vi "XNET Example IP Stack Config - Add Proxy Server Extended.vi"(0 "config in":string, 1 "forwarding destination address":string, 2 "forwarding destination port":u16, 5 "protocol":string(combo)="tcp", 7 "direction":string(combo)="outbound", 9 "listen port":u16, 11 "error in (no error)":errorcluster, 12 "listen address":string, 13 "forwarding source address":string, 14 "forwarding source port":u16) -> (4 "config out":string, 15 "error out":errorcluster)   [LabVIEW 2026]
doc: "This example subVI adds configuration for a single proxy server instance to an existing JSON configuration string for use with XNET IP Stack Create.vi. Configuration parameter definitions:\n\nprotocol: Protocol to use for the proxy server, which can be one of 1) tcp, 2) udp.\n\ndirection: Direction to use for the proxy server, which can be one of 1) outbound, 2) inbound. When using TCP, this specifies the direction of the TCP connection. Once connected, TCP communication is always bidirectional through a single proxy server. When using UDP, this specifies the direction of communication, which is always unidirectional. Use two proxy servers if you require bidirectional UDP communication.\n\nlisten address: The proxy server listens for data on this address. This can be 'any', 'localhost', or a valid IPv4 or IPv6 address using standard IETF syntax. This property is optional; if not provided or if set to an empty string, outbound servers use the default value 'localhost', and inbound servers use the default value 'any'.\n\nlisten port: The proxy server listens for data on this port. Values from 1-65535 identify a valid port number.\n\nforwarding destination address: The proxy server forwards all received data to this address. This can be 'localhost' or a valid IPv4 or IPv6 address using standard IETF syntax.\n\nforwarding destination port: The proxy server forwards all received data to this port. Values from 1-65535 identify a valid port number.\n\nforwarding source address: The proxy server forwards all data using this source address. This can be 'any', 'localhost', or a valid IPv4 or IPv6 address using standard IETF syntax. This property is optional; if not provided or if set to an empty string, the default value 'any' is used.\n\nforwarding source port: The proxy server forwards all data using this source port. Values from 0-65535 identify a valid port number. This property is optional; if not provided, the default value 0 is used, which assigns a randomly-selected port.\n\nYou can re-use this subVI in one of two ways: a) copy the subVI from the example diagram to your VI diagram, which re-uses the subVI unchanged (located in the XNET library), or b) use Save As to create a copy of the subVI in your application folder, and change as needed."
uses:
  XNET Example IP Stack Config - Stack Extended.ctl
  <vilib>/xnet/xnet.llb/XNET Example IP Stack Config - XNET Interface.ctl
  <vilib>/xnet/xnet.llb/XNET Example IP Stack Config - MAC.ctl
  <vilib>/xnet/xnet.llb/XNET Example IP Stack Config - VLAN.ctl
  <vilib>/xnet/xnet.llb/XNET Example IP Stack Config - Static Address.ctl
  <vilib>/xnet/xnet.llb/XNET Example IP Stack Config - Static IPv6 Address.ctl
  XNET Example IP Stack Config - Proxy Server Extended.ctl
  79557c27-0234-40f6-b19b-098455816367.vi
  9d5c5eb7-7114-4a22-bbf1-c987cc0edc55.vi
  <vilib>/JDP Science/JSONtext/JSON text to Variant (path).vi
  <vilib>/JDP Science/JSONtext/Find Item.vi
  <vilib>/JDP Science/JSONtext/Next JSON Value.vi
  <vilib>/JDP Science/JSONtext/String Subset.vi
  <vilib>/JDP Science/JSONtext/Parsing/Advance past next JSON Value (inlined COPY).vi
  <vilib>/JDP Science/JSONtext/Parsing/Advance past whitespace.vi
  <vilib>/JDP Science/JSONtext/Parsing/Advance past String.vi
  <vilib>/JDP Science/JSONtext/Parsing/Advance past Number.vi
  <vilib>/JDP Science/JSONtext/Parsing/Advance past Line Ending.vi
  <vilib>/Utility/Data Type/Get Type Information.vi
  <vilib>/JDP Science/JSONtext/JSON text to Variant.vi
  <vilib>/JDP Science/JSONtext/Parsing/Parse Full Path or Item Name.vi
  <vilib>/JDP Science/JSONtext/Parsing/Advance past Array.vi
  <vilib>/JDP Science/JSONtext/Parsing/Advance past Object.vi
  <vilib>/JDP Science/JSONtext/support/Error Cluster From Code.vi
  <vilib>/JDP Science/JSONtext/Offset/Find Item Locations by Path.vi
  <vilib>/JDP Science/JDP Science Common Utilities/Array of Variants to Cluster.vi
  <vilib>/JDP Science/JSONtext/LVClass Serializer/JSONtext LVClass Serializer.lvclass
  <vilib>/addons/_JKI.lib/Serialization/JSON/JKI JSON Serialization.lvlib
panel:
  out "Variant":variant
  out "error out 3":errorcluster
  in  "error in":errorcluster
  out "Cluster":T1={"schema"="", "xnetInterfaces"=[{"name"="", "MACs"=[{"address"="", "VLANs"=[{"name"="", "isTagged"=FALSE, "id"=0, "priority"=0, "IPv4"={"mode"="static", "staticAddresses"=[]}, "IPv6"={"mode"="", "staticAddresses"=[]}, "staticArpTable"=[]}]}], "staticArpTable"=[]}], "proxyServers"=[]}
  out "error out 2":errorcluster
  in  "error in (no error) 2":errorcluster
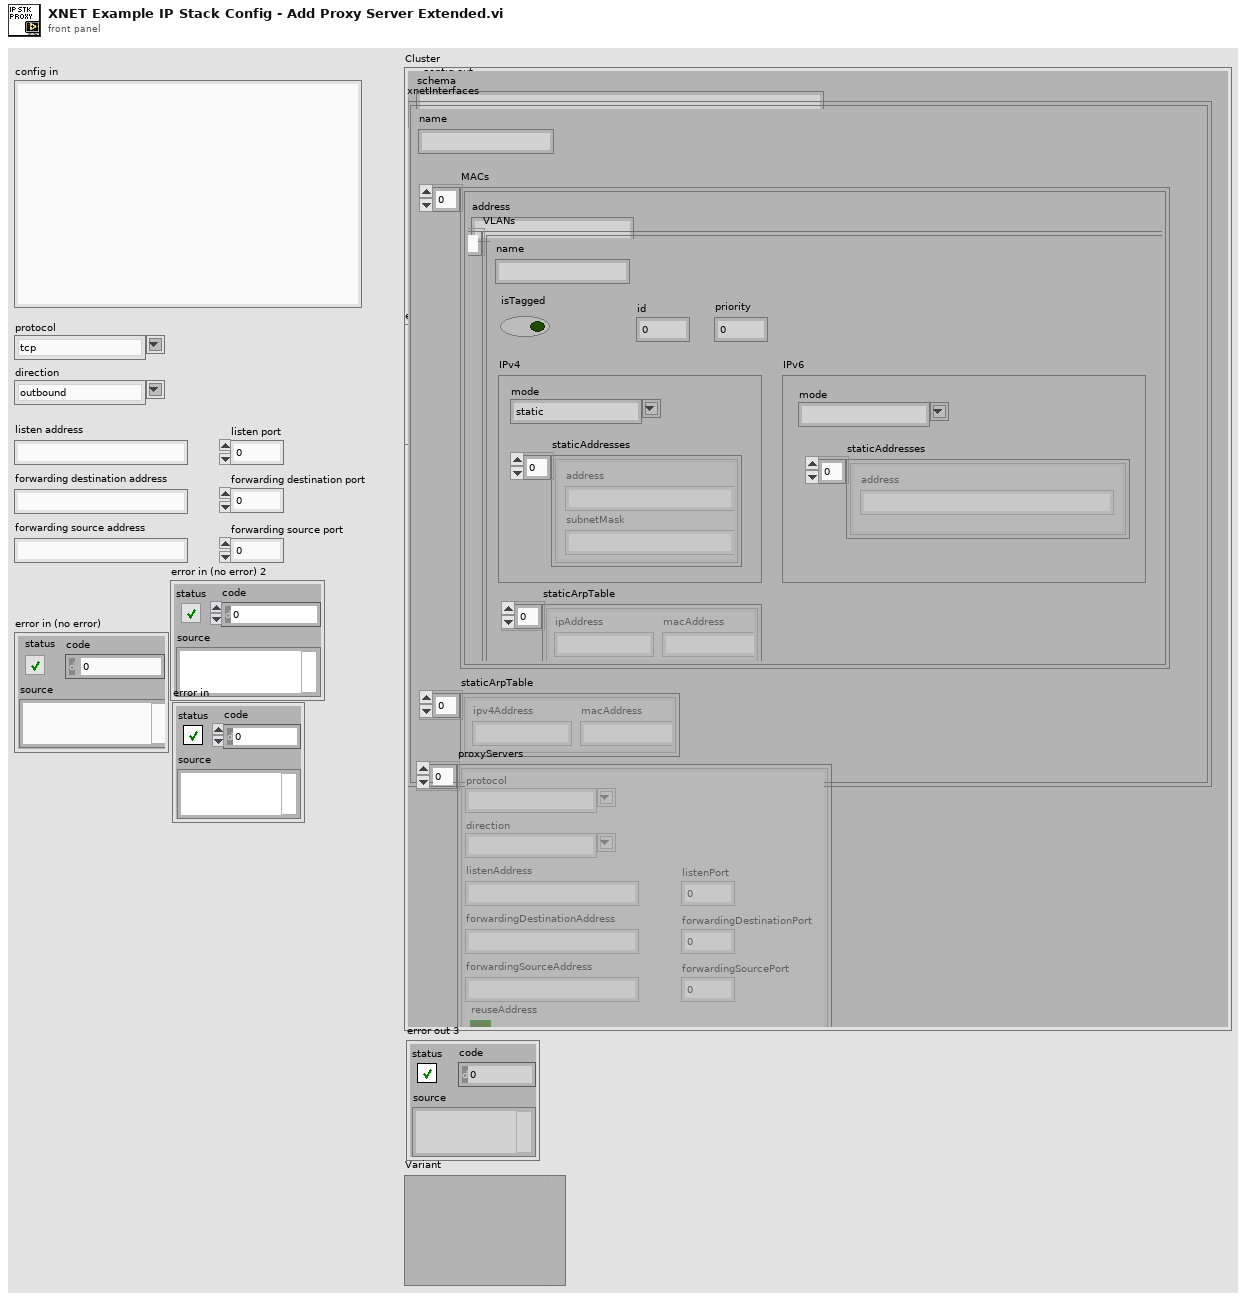
[diagram p1: front panel]
types:
  T1 = typedef "XNET Example IP Stack Config - Stack Extended.ctl" = cluster{"schema":string, "xnetInterfaces":T2[], "proxyServers":T7[]}
  T2 = typedef "XNET Example IP Stack Config - XNET Interface.ctl" = cluster{"name":string, "MACs":T3[], "staticArpTable":cluster{"ipv4Address":string, "macAddress":string}[]}
  T3 = typedef "XNET Example IP Stack Config - MAC.ctl" = cluster{"address":string, "VLANs":T4[]}
  T4 = typedef "XNET Example IP Stack Config - VLAN.ctl" = cluster{"name":string, "isTagged":bool, "id":u16, "priority":u8, "IPv4":cluster{"mode":string, "staticAddresses":T5[]}, "IPv6":cluster{"mode":string, "staticAddresses":T6[]}, "staticArpTable":cluster{"ipAddress":string, "macAddress":string}[]}
  T5 = typedef "XNET Example IP Stack Config - Static Address.ctl" = cluster{"address":string, "subnetMask":string}
  T6 = typedef "XNET Example IP Stack Config - Static IPv6 Address.ctl" = cluster{"address":string}
  T7 = typedef "XNET Example IP Stack Config - Proxy Server Extended.ctl" = cluster{"protocol":string, "direction":string, "listenAddress":string, "listenPort":u16, "forwardingDestinationAddress":string, "forwardingDestinationPort":u16, "forwardingSourceAddress":string, "forwardingSourcePort":u16, "reuseAddress":bool}
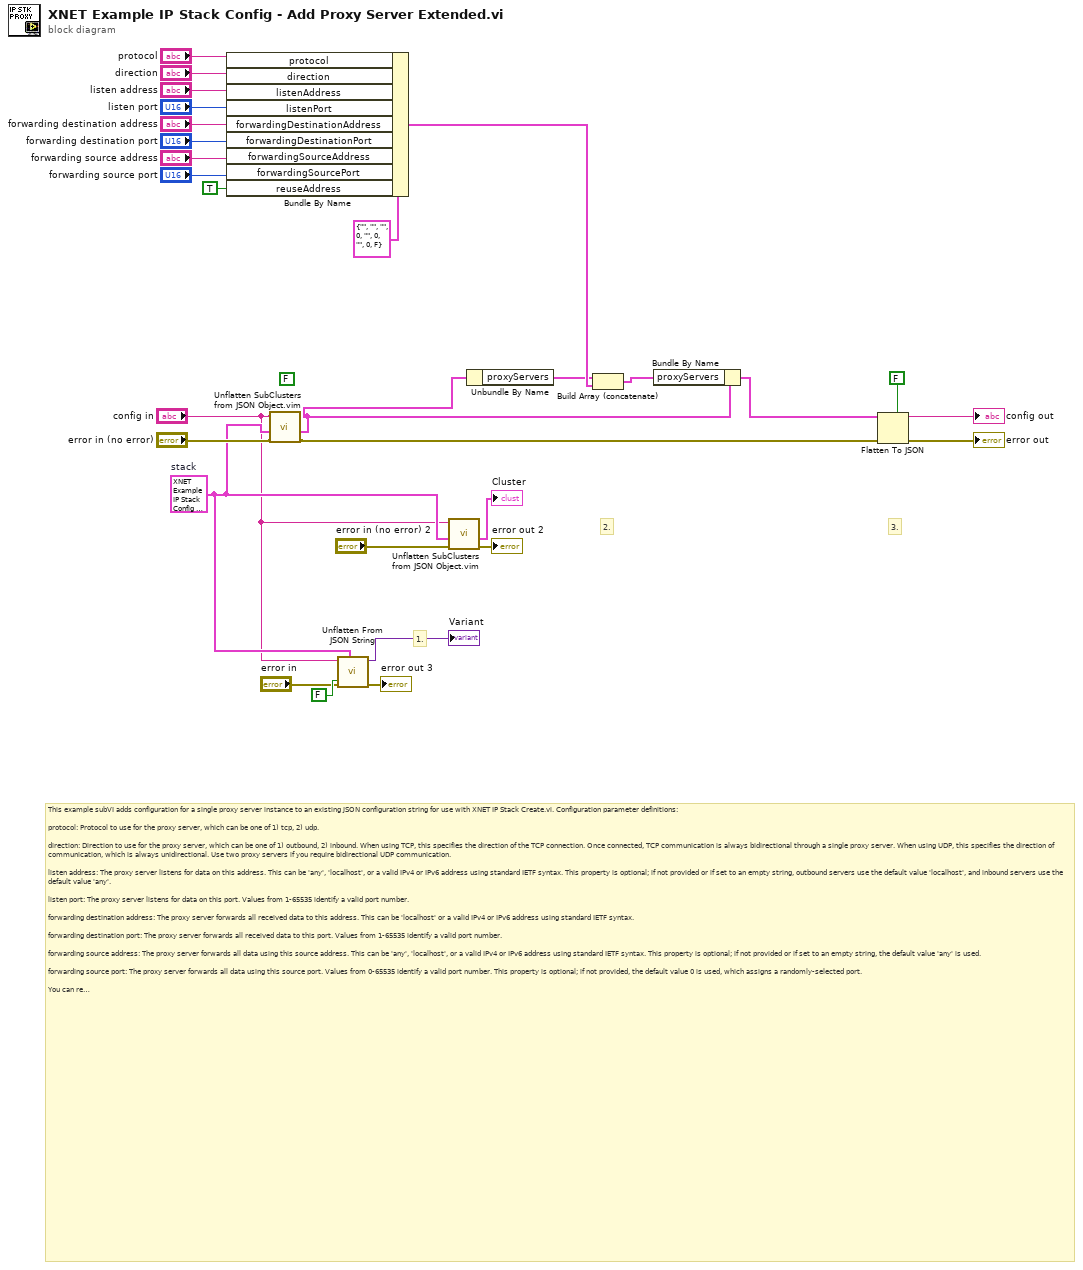
[diagram p0: block diagram]
diagram:
  (unwired) FALSE ("enable LabVIEW extensions? (T)")
  w4 = T1 {"schema"="", "xnetInterfaces"=[{"name"="", "MACs"=[{"address"="", "VLANs"=[{"name"="", "isTagged"=FALSE, "id"=0, "priority"=0, "IPv4"={"mode"="static", "staticAddresses"=[]}, "IPv6"={"mode"="", "staticAddresses"=[]}, "staticArpTable"=[]}]}], "staticArpTable"=[]}], "proxyServers"=[]}  # stack
  # "3."
  # "2."
  # "1."
  # "This example subVI adds configuration for a single proxy server instance to an existing JSON configuration string for use with XNET IP Stack Create.vi. Configuration parameter definitions:\n\nprotocol: Protocol to use for the proxy server, which can be one of 1) tcp, 2) udp.\n\ndirection: Direction to use for the proxy server, which can be one of 1) outbound, 2) inbound. When using TCP, this specifies the direction of the TCP connection. Once connected, TCP communication is always bidirectional through a single proxy server. When using UDP, this specifies the direction of communication, which is always unidirectional. Use two proxy servers if you require bidirectional UDP communication.\n\nlisten address: The proxy server listens for data on this address. This can be 'any', 'localhost', or a valid IPv4 or IPv6 address using standard IETF syntax. This property is optional; if not provided or if set to an empty string, outbound servers use the default value 'localhost', and inbound servers use the default value 'any'.\n\nlisten port: The proxy server listens for data on this port. Values from 1-65535 identify a valid port number.\n\nforwarding destination address: The proxy server forwards all received data to this address. This can be 'localhost' or a valid IPv4 or IPv6 address using standard IETF syntax.\n\nforwarding destination port: The proxy server forwards all received data to this port. Values from 1-65535 identify a valid port number.\n\nforwarding source address: The proxy server forwards all data using this source address. This can be 'any', 'localhost', or a valid IPv4 or IPv6 address using standard IETF syntax. This property is optional; if not provided or if set to an empty string, the default value 'any' is used.\n\nforwarding source port: The proxy server forwards all data using this source port. Values from 0-65535 identify a valid port number. This property is optional; if not provided, the default value 0 is used, which assigns a randomly-selected port.\n\nYou can re-use this subVI in one of two ways: a) copy the subVI from the example diagram to your VI diagram, which re-uses the subVI unchanged (located in the XNET library), or b) use Save As to create a copy of the subVI in your application folder, and change as needed.\n1. Use the LabVIEW Unflatten From JSON VI to generate a stack configuration cluster from the JSON configuration string.\n    Since the XNET IP stack JSON is intended to support non-LabVIEW code, avoid LabVIEW-only extensions.\n2. Form a single proxy server configuration and add it to the stack configuration.\n3. Use the LabVIEW Flatten to JSON VI to generate the string from the arrays and clusters.\n    Since the XNET IP stack JSON is intended to support non-LabVIEW code, avoid LabVIEW-only extensions."
  n1 = Bundle By Name(cluster=T7 {"protocol"="", "direction"="", "listenAddress"="", "listenPort"=0, "forwardingDestinationAddress"="", "forwardingDestinationPort"=0, "forwardingSourceAddress"="", "forwardingSourcePort"=0, "reuseAddress"=FALSE} ("proxyServers"), "protocol"="protocol", "direction"="direction", "listenAddress"="listen address", "listenPort"="listen port", "forwardingDestinationAddress"="forwarding destination address", "forwardingDestinationPort"="forwarding destination port", "forwardingSourceAddress"="forwarding source address", "forwardingSourcePort"="forwarding source port", "reuseAddress"=TRUE) -> (w15:T7)
  n2 = call "Unflatten SubClusters from JSON Object.vim"("error in (no error)"="error in (no error)", "Any Cluster"=w4, "JSON"="config in") -> ("error out"=w1:errorcluster, "Cluster"=w2:T1)  [unwired: 7 in]
  n3 = call <vilib>:"Unflatten From JSON String.vi"("Nulls as Defaults (F)"=FALSE, "Type and Defaults"=w4, "error in"="error in", "JSON String"="config in") -> ("error out"=→"error out 3":errorcluster, "Variant"=→"Variant":variant)  [unwired: 6 in]
  n4 = call "Unflatten SubClusters from JSON Object.vim"("error in (no error)"="error in (no error) 2", "Any Cluster"=w4, "JSON"="config in") -> ("error out"=→"error out 2":errorcluster, "Cluster"=→"Cluster":T1)  [unwired: 7 in]
  n5 = Unbundle By Name(w2) -> ("proxyServers"=w7:T7[])
  n6 = Build Array (concatenate)(w7, w15) -> (w6:T7[])
  n7 = Bundle By Name(cluster=w2, "proxyServers"=w6) -> (w19:T1)
  n8 = Flatten To JSON(enable LabVIEW extensions? (T)=FALSE, anything=w19, error in (no error)=w1) -> (JSON string=→"config out":string, 11:→"error out":errorcluster)
